vi "Network Command Engine.vi"(8 "error in (no error)":errorcluster, 10 "Parameters":T1 {"Config"."Industrial Settings"."Write Refs"."Data Reference" format="%.0x"; "Config"."Industrial Settings"."Read Refs"."Data Reference" format="%.0x"; "Config"."PID Settings"."Read Refs"."Data Reference" format="%.0x"; "Config"."PID Settings"."Write Refs"."Data Reference" format="%.0x"}, 11 "State Variables":T9) -> (0 "error out":errorcluster)   [LabVIEW 2013, in "Control Addon Engine.lvlib" / "Network Common API.lvlib"]
uses:
  Network Common API.lvlib
  Inline Async API/Controls/Engine State Variables.ctl
  TCP Refs.ctl
  Network Comm Global Ref.ctl
  Stop FG/Stop Global Ref.ctl
  Types/RT Configuration.ctl
  Shared/Types/Gain Schedule.ctl
  Shared/Types/Compiled Settings.ctl
  Shared/Types/Compiled PID Settings.ctl
  <vilib>/NI Veristand/Custom Device API/Block Data Reference.ctl
  <vilib>/NI Veristand/Custom Device API/Data Reference.ctl
  Shared/Types/Compiled Industrial Settings.ctl
  Shared/Types/Compiled Industrial Parameters.ctl
  <userlib>/STM/Connection Manager/TCP/stm_TCPConnectionMethod.ctl
  Stop FG/Stop Global Commands.ctl
  <userlib>/STM/TCP/stm_TCP Read Options.ctl
  Shared/Types/Update Parameters Message.ctl
  <userlib>/STM/TCP/STM Read Message (TCP).vi
  <userlib>/STM/TCP/STM Write Message (TCP).vi
  <vilib>/NI Veristand/Custom Device Tools/Custom Device Utility Library/NI VeriStand - Print Debug String.vi
  <userlib>/STM/TCP/STM Get Connection Reference (TCP).vi
  Stop FG/Stop FG.lvlib
  Shared/Control Addon Shared.lvlib
  Control Addon Engine.lvlib
  Inline Async API/Inline Async API.lvlib
  <vilib>/NI Veristand/Custom Device API/Custom Device API.lvlib
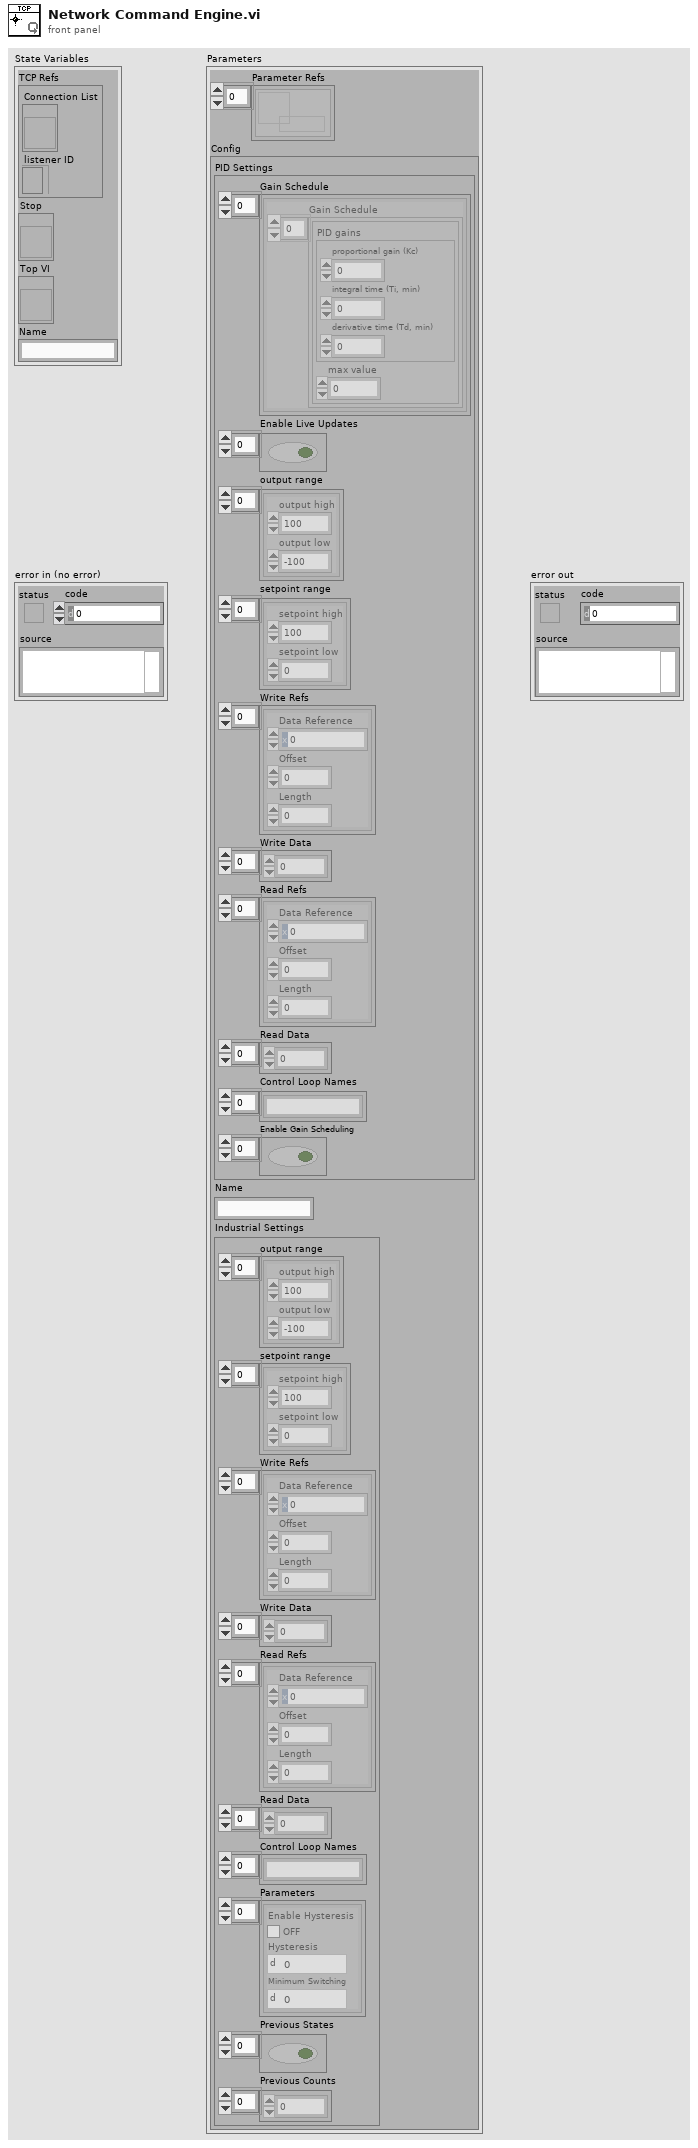
[diagram p1: front panel]
types:
  T1 = typedef "Control Addon Engine.lvlib/RT Configuration.ctl" = cluster{"Parameter Refs":refnum<data-value>[], "Config":T2}
  T2 = typedef "Control Addon Shared.lvlib/Compiled Settings.ctl" = cluster{"PID Settings":T3, "Name":string, "Industrial Settings":T7}
  T3 = typedef "Control Addon Shared.lvlib/Compiled PID Settings.ctl" = cluster{"Gain Schedule":T4[], "Enable Live Updates":bool[], "output range":cluster{"output high":dbl, "output low":dbl}[], "setpoint range":cluster{"setpoint high":dbl, "setpoint low":dbl}[], "Write Refs":T5[], "Write Data":dbl[], "Read Refs":T5[], "Read Data":dbl[], "Control Loop Names":string[], "Enable Gain Scheduling":bool[]}
  T4 = typedef "Control Addon Shared.lvlib/Gain Schedule.ctl" = cluster{"Gain Schedule":cluster{"PID gains":cluster{"proportional gain (Kc)":dbl, "integral time (Ti, min)":dbl, "derivative time (Td, min)":dbl}, "max value":dbl}[]}
  T5 = typedef "Custom Device API.lvlib/Block Data Reference.ctl" = cluster{"Data Reference":T6, "Offset":i32, "Length":i32}
  T6 = typedef "Custom Device API.lvlib/Data Reference.ctl" = i32
  T7 = typedef "Control Addon Shared.lvlib/Compiled Industrial Settings.ctl" = cluster{"output range":cluster{"output high":dbl, "output low":dbl}[], "setpoint range":cluster{"setpoint high":dbl, "setpoint low":dbl}[], "Write Refs":T5[], "Write Data":dbl[], "Read Refs":T5[], "Read Data":dbl[], "Control Loop Names":string[], "Parameters":T8[], "Previous States":bool[], "Previous Counts":u64[]}
  T8 = typedef "Control Addon Shared.lvlib/Compiled Industrial Parameters.ctl" = cluster{"Enable Hysteresis":bool, "Hysteresis":dbl, "Minimum Switching":u64}
  T9 = typedef "Control Addon Engine.lvlib/Inline Async API.lvlib/Engine State Variables.ctl" = cluster{"TCP Refs":T10, "Stop":T12, "Top VI":refnum<vi>, "Name":string}
  T10 = typedef "Control Addon Engine.lvlib/Network Common API.lvlib/TCP Refs.ctl" = cluster{"Connection List":T11, "listener ID":refnum<k5>}
  T11 = typedef "Control Addon Engine.lvlib/Network Common API.lvlib/Network Comm Global Ref.ctl" = refnum<vi>
  T12 = typedef "Control Addon Engine.lvlib/Stop FG.lvlib/Stop Global Ref.ctl" = refnum<vi>
  T13 = typedef "Control Addon Engine.lvlib/Stop FG.lvlib/Stop Global Commands.ctl" = enum16{"Write", "Read", "Reset"}
  T14 = typedef "stm_TCPConnectionMethod.ctl" = enum16{"Initialize", "Add Connection", "Set Properties", "Get Connection(s)", "Remove Connection", "Remove All Connections", "Get Connection Count"}
  T15 = typedef "Control Addon Shared.lvlib/Update Parameters Message.ctl" = cluster{"Control Loop":string, "Gain Schedule":cluster{"PID gains":cluster{"proportional gain (Kc)":dbl, "integral time (Ti, min)":dbl, "derivative time (Td, min)":dbl}, "max value":dbl}[]}
  T16 = typedef "stm_TCP Connection Info.ctl" = cluster{"connection ID":refnum<k5>, "Meta data":T17[]}
  T17 = typedef "stm_MetaDataElement.ctl" = string
  T18 = typedef "stm_TCP Read Options.ctl" = cluster{"Ignore Timeout Error":bool, "timeout ms (1000)":i32}
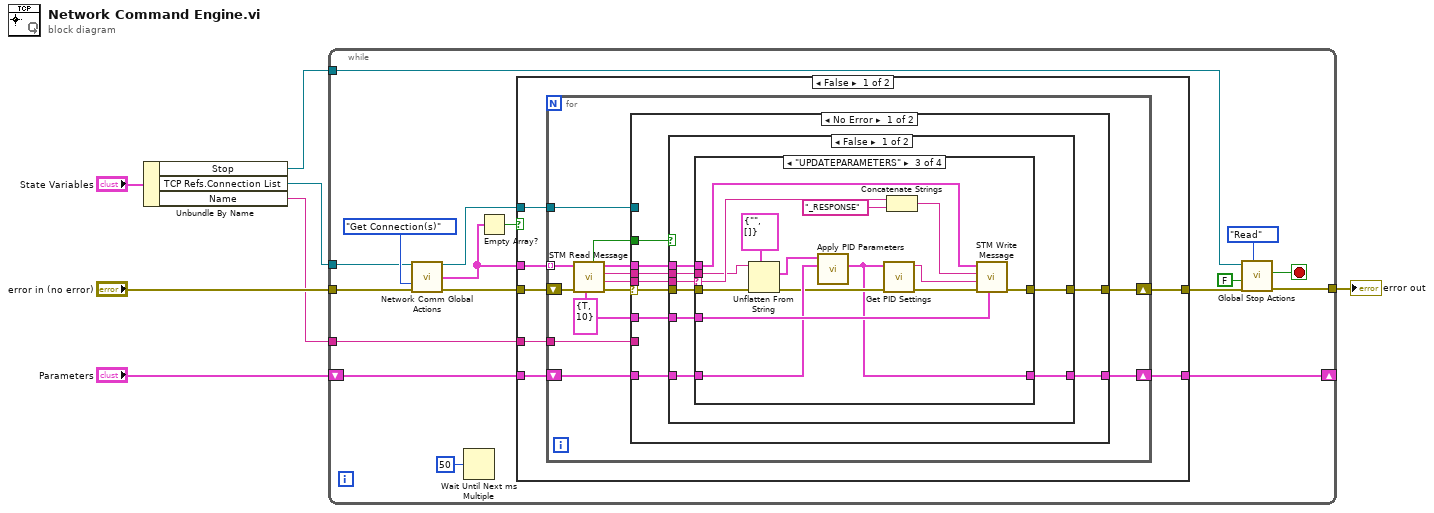
[diagram p0: block diagram]
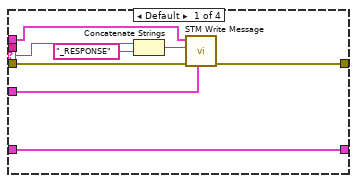
[diagram p2: hidden frame]
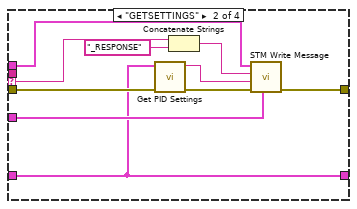
[diagram p3: hidden frame]
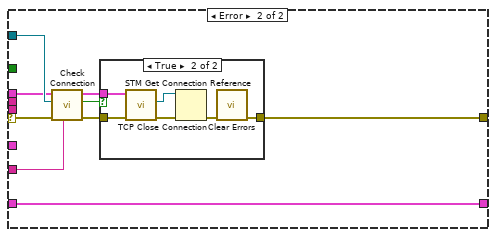
[diagram p6: hidden frame]
diagram:
  n1 = Unbundle By Name("State Variables") -> ("Stop"=w7:T12, "TCP Refs.Connection List"=w5:T11, "Name"=w2:string)
  n2 = while {
    tunnel: "error in (no error)" -> [w20]
    tunnel: [w10] -> w3
    tunnel: w5 -> [w14]
    tunnel: w7 -> [w13]
    tunnel: w2 -> [w12]
    shift-right: [w8] -> _
    shift-left: "Parameters" -> [w9]
    stop <- w15 stop-if-true
    n3 = call "Network Comm Global Actions.vi"("ref in"=w14, "Method"=stm_TCPConnectionMethod."Get Connection(s)", "error in (no error)"=w20) -> ("ref out"=w18:T11, "All Connections"=w21:T16[], "error out"=w19:errorcluster)  [unwired: 6 in, 4 out]
    n4 = Wait Until Next ms Multiple(millisecond multiple=u32 50 ("STM Update Rate")) -> ()  [unwired: 1 out]
    n5 = Empty Array?(array=w21) -> (empty?=w22:bool)
    n6 = case shown="False" w22 {
      tunnel: w21 -> [w31 _]
      tunnel: w19 -> [w27 w116]
      tunnel: w18 -> [w30 _]
      tunnel: [w29 w116] -> w16
      tunnel: w12 -> [w28 _]
      tunnel: w9 -> [w26 w115]
      tunnel: [w25 w115] -> w8
      frame False {
        n7 = for {
          tunnel: w31 -> [w40] mode=indexing
          tunnel: w30 -> [w44]
          shift-right: [w43] -> w29
          shift-left: w27 -> [w42]
          tunnel: w28 -> [w34]
          shift-right: [w32] -> w25
          shift-left: w26 -> [w33]
          w35 = T18 {"Ignore Timeout Error"=TRUE, "timeout ms (1000)"=10} ("options")
          n8 = call-poly <userlib>:"STM Read Message.vi"("Options"=w35, "error in"=w42, "Connection Info"=w40) -> ("error out"=w41:errorcluster, "Name"=w37:T17, "data string"=w38:string, "Connection Info Out"=w39:T16, "Timed Out?"=w36:bool)  [unwired: 3 in, 1 out]
          n9 = case shown="No Error" w41 {
            selector: w41 -> [w53 w102]
            tunnel: w44 -> [_ w104]
            tunnel: w39 -> [w48 w103]
            tunnel: [w52 w101] -> w43
            tunnel: w38 -> [w51 _]
            tunnel: w37 -> [w50 _]
            tunnel: w36 -> [w49 _]
            tunnel: w35 -> [w47 _]
            tunnel: w34 -> [_ w100]
            tunnel: w33 -> [w46 w99]
            tunnel: [w45 w99] -> w32
            frame No Error {
              n10 = case shown="False" w49 {
                tunnel: w53 -> [w59 w98]
                tunnel: [w61 w98] -> w52
                tunnel: w51 -> [w57 _]
                tunnel: w50 -> [w58 _]
                tunnel: w48 -> [w60 _]
                tunnel: w47 -> [w56 _]
                tunnel: w46 -> [w55 w97]
                tunnel: [w54 w97] -> w45
                frame False {
                  n11 = case shown="\"UPDATEPARAMETERS\"" w58 {
                    selector: w58 -> [w66 w76 w91 _]
                    tunnel: w59 -> [w63 w73 w88 w96]
                    tunnel: [w69 w79 w94 w96] -> w61
                    tunnel: w57 -> [_ _ w85 _]
                    tunnel: w60 -> [w68 w78 w93 _]
                    tunnel: w56 -> [w64 w74 w89 _]
                    tunnel: w55 -> [w62 w70 w87 w95]
                    tunnel: [w62 w70 w80 w95] -> w54
                    frame Default {
                      n12 = Concatenate Strings(w66, "_RESPONSE" ("string")) -> (w65:string)
                      n13 = call-poly <userlib>:"STM Write Message.vi"("Options"=w64, "error in (no error)"=w63, "Name"=w65, "Connection Info"=w68) -> ("error out"=w69:errorcluster)  [unwired: 6 in, 1 out]
                    }
                    frame "GETSETTINGS" {
                      n14 = call "Get PID Settings.vi"("error in (no error)"=w73, "Parameters"=w70) -> ("error out"=w72:errorcluster, "Flattened String"=w71:string)  [unwired: 8 in]
                      n15 = Concatenate Strings(w76, "_RESPONSE" ("string")) -> (w75:string)
                      n16 = call-poly <userlib>:"STM Write Message.vi"("Options"=w74, "error in (no error)"=w72, "Data"=w71, "Name"=w75, "Connection Info"=w78) -> ("error out"=w79:errorcluster)  [unwired: 5 in, 1 out]
                    }
                    frame "UPDATEPARAMETERS" {
                      n17 = Unflatten From String(type=T15 {"Control Loop"="", "Gain Schedule"=[]}, binary string=w85, error in (no error)=w88) -> (value=w84:T15, error out=w81:errorcluster)  [unwired: 2 in, 1 out]
                      n18 = call "Apply PID Parameters.vi"("Parameters in"=w87, "UpdateParameters"=w84) -> ("Parameters out"=w80:T1)  [unwired: 9 in]
                      n19 = call "Get PID Settings.vi"("error in (no error)"=w81, "Parameters"=w80) -> ("error out"=w82:errorcluster, "Flattened String"=w83:string)  [unwired: 8 in]
                      n20 = Concatenate Strings(w91, "_RESPONSE" ("string")) -> (w90:string)
                      n21 = call-poly <userlib>:"STM Write Message.vi"("Options"=w89, "error in (no error)"=w82, "Data"=w83, "Name"=w90, "Connection Info"=w93) -> ("error out"=w94:errorcluster)  [unwired: 5 in, 1 out]
                    }
                    frame "" {
                    }
                  }
                }
                frame True {
                }
              }
            }
            frame Error {
              n22 = call "Check Connection.vi"("Name"=w100, "error in (no error)"=w102, "ref in"=w104, "Connection In"=w103) -> ("error out"=w107:errorcluster, "Disconnected"=w105:bool, "Connection In"=w106:T16)  [unwired: 5 in]
              n23 = case shown="True" w105 {
                tunnel: [w108 w111] -> w101
                tunnel: w107 -> [w108 w114]
                tunnel: w106 -> [_ w109]
                frame False {
                }
                frame True {
                  n24 = call-poly <userlib>:"STM Get Connection Reference.vi"("error in"=w114, "Connection Info"=w109) -> ("error out"=w113:errorcluster, "connection ID out"=w112:refnum<k5>)  [unwired: 7 in, 1 out]
                  n25 = TCP Close Connection(connection ID=w112, error in (no error)=w113) -> (error out=w110:errorcluster)  [unwired: 1 in, 1 out]
                  n26 = call <vilib>:"Clear Errors.vi"("error in (no error)"=w110) -> ("error out"=w111:errorcluster)  [unwired: 6 in]
                }
              }
            }
          }
        }
      }
      frame True {
      }
    }
    n27 = call "Global Stop Actions.vi"("Command"=Stop_Global_Commands."Read", "error in (no error)"=w16, "Stop on Error?"=FALSE, "vi reference"=w13) -> ("error out"=w10:errorcluster, "Latched Stop"=w15:bool)  [unwired: 5 in, 1 out]
  }
  "error out" <- w3
